vi "New Message.vi"(8 "error in (no error)":errorcluster, 11 "Chat Room Model in":refnum<class "Chat Window Model.lvclass">) -> (0 "error out":errorcluster, 3 "Chat Room Model out":refnum<class "Chat Window Model.lvclass">)   [LabVIEW 2020, in "Chat Room Model.lvlib" / "Chat Window Model.lvclass"]
uses:
  Chat Window Model.lvclass
  Chat Window Model.lvclass/Chat Window Model.ctl
  Chat Window UI Controller/Chat Window Controller Messages/Update Message Log Msg/Update Message Log Msg.lvclass
panel:
  in  "New Message":string
  in  "From":string
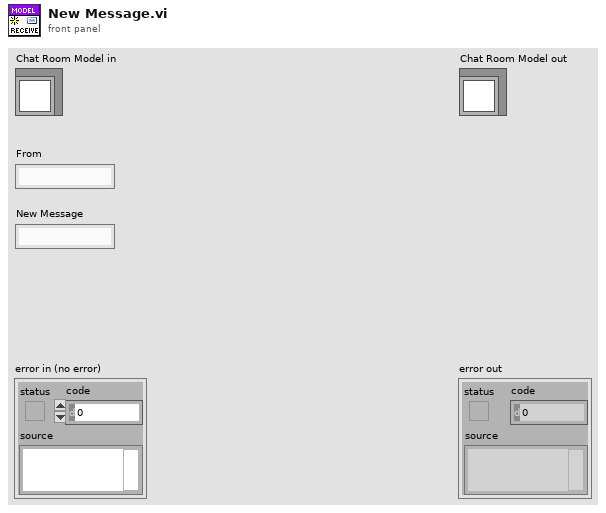
[diagram p1: front panel]
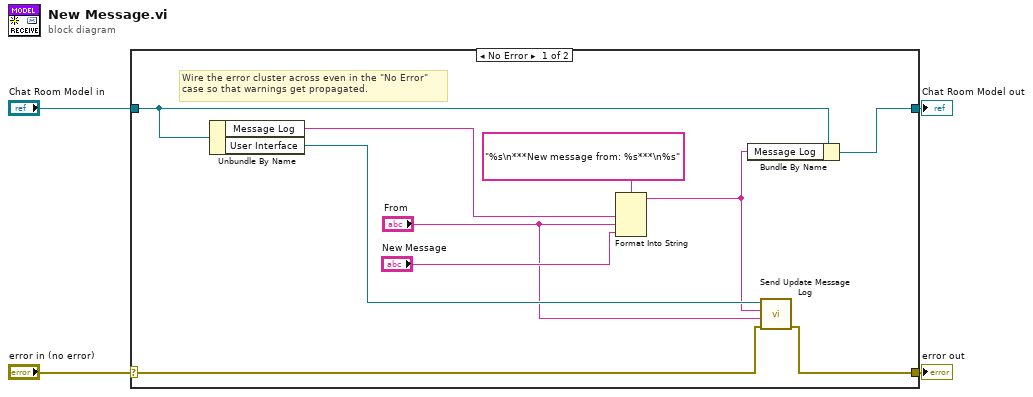
[diagram p0: block diagram]
diagram:
  n1 = case shown="No Error" "error in (no error)" {
    selector: "error in (no error)" -> [w6 w16]
    tunnel: [w5 w16] -> w3
    tunnel: [w10 w15] -> w1
    tunnel: "Chat Room Model in" -> [w11 w15]
    frame No Error {
      # "Wire the error cluster across even in the \"No Error\"\ncase so that warnings get propagated."
      n2 = Unbundle By Name(w11) -> ("Message Log"=w12:string, "User Interface"=w14:refnum<class "Message Enqueuer.lvclass">)
      n3 = Format Into String(format string="%s\n***New message from: %s***\n%s", w12, "From", "New Message") -> (resulting string=w8:string)  [unwired: 2 in, 1 out]
      n4 = Bundle By Name(cluster=w11, "Message Log"=w8) -> (w10:refnum<class "Chat Window Model.lvclass">)
      n5 = call "Send Update Message Log.vi"("error in (no error)"=w6, "From"="From", "Newl Msg"=w8, "Message Enqueuer"=w14) -> ("error out"=w5:errorcluster)  [unwired: 7 in]
    }
    frame Error {
    }
  }
  "error out" <- w3
  "Chat Room Model out" <- w1
